vi "Make_Different_Variants_of_Tracks-5.vi"(8 "error IN":errorcluster, 9 "[IN] # of Longest track\nInside the Group of Tracks":i32, 10 "[IN] Index of Earliest \nProblem Point Inside":i32, 11 "[IN] Still connected\ntracks in group":T2) -> (0 "error OUT":errorcluster, 1 "[OUT] Special case!":bool, 3 "[OUT] Subtracks":T1(array[cluster]))   [LabVIEW 2013]
doc: "The subVI formates competing subtracks \nTwo cases are considered: \nSplitting event => only variants after splitting + account the origin of one of subtracks\nMerging event => competition between different variants of elongations"
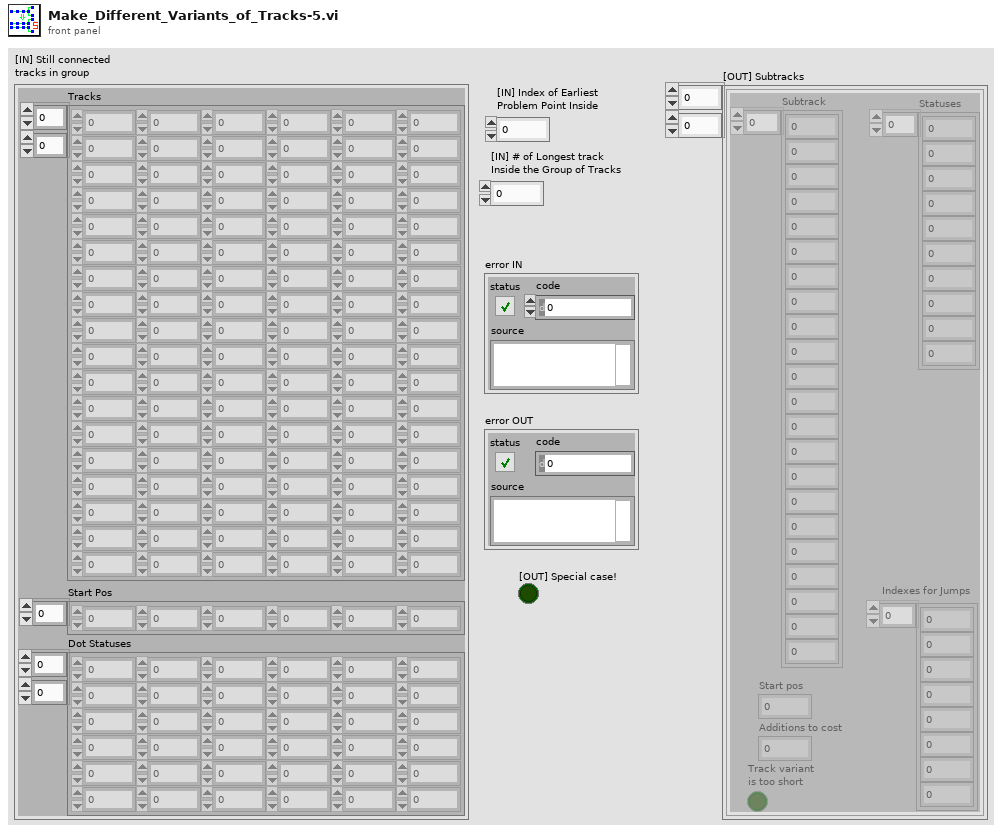
[diagram p1: front panel]
types:
  T1 = cluster{"Subtrack":dbl[], "Statuses":i16[], "Start pos":i32, "Additions to cost":i32, "Track variant \nis too short":bool, "Indexes for Jumps":i32[]}[][]
  T2 = cluster{"Tracks":dbl[][], "Start Pos":i32[], "Dot Statuses":i16[][]}
  T3 = cluster{"Subtrack":dbl[], "Statuses":i16[], "Start pos":i32, "Additions to cost":i32, "Track variant \nis too short":bool, "Indexes for Jumps":i32[]}
  T4 = cluster{"Subtrack":dbl[], "Statuses":i16[], "Start pos":i32, "Additions to cost":i32, "Track variant \nis too short":bool, "Indexes for Jumps":i32[]}[]
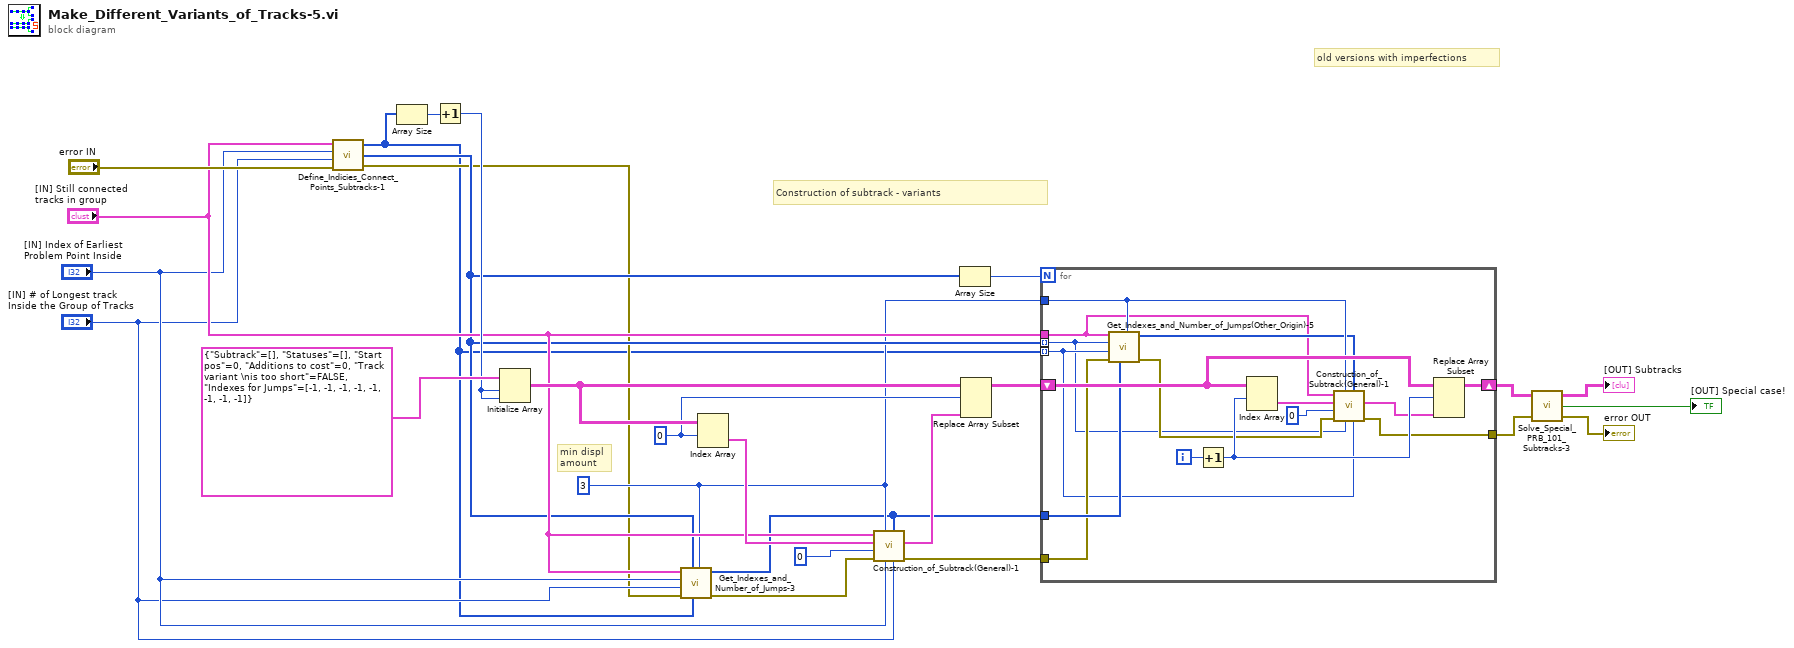
[diagram p0: block diagram]
diagram:
  w20 = 0
  w7 = 3 ("[IN] Minimal Subtrack Length \n(Points without problems) for\nMaking Desicion")
  # "old versions with imperfections"
  # "min displ \namount"
  # "Construction of subtrack - variants"
  n1 = call "Define_Indicies_Connect_Points_Subtracks-1.vi"("error IN"="error IN", "[IN] Index of track with\n(problem displacement)"="[IN] # of Longest track\nInside the Group of Tracks", "[IN] Index of problem\ndisplacement inside track"="[IN] Index of Earliest \nProblem Point Inside", "[IN] Track group"="[IN] Still connected\ntracks in group") -> ("error OUT"=w4:errorcluster, "[OUT] Index of \nconnected dots\ninside the track"=w8:i32[], "[OUT] Index of connected\ntracks with problem dot"=w3:i32[])
  n2 = Array Size(array=w3) -> (size(s)=w25:i32)
  n3 = Increment(x=w25) -> (x+1=w16:i32)
  n4 = Initialize Array(T3 {"Subtrack"=[], "Statuses"=[], "Start pos"=0, "Additions to cost"=0, "Track variant \nis too short"=FALSE, "Indexes for Jumps"=[-1, -1, -1, -1, -1, -1, -1, -1]}, w16, w16) -> (w23:T1)
  n5 = call "Get_Indexes_and_Number_of_Jumps-3.vi"("[IN] Minimal Subtrack\nLength for Making Desicion"=w7, "[IN] Index of connected\ntracks with problem dot"=w3, "[IN] Index of connected \ndots inside the track"=w8, "error IN"=w4, "[IN] # of Track with\nFirst Problem Point"="[IN] # of Longest track\nInside the Group of Tracks", "[IN] Index of First Pro\nblem Point Inside Track"="[IN] Index of Earliest \nProblem Point Inside", "[IN] Still connected\ntracks in group"="[IN] Still connected\ntracks in group") -> ("error OUT"=w2:errorcluster, "[OUT] Indexes for Jumps"=w1:i32[])  [unwired: 1 in, 1 out]
  n6 = Index Array(array=w23, index (row)=w20) -> (element=w22:T4)  [unwired: 1 in]
  n7 = call "Construction_of_Subtrack(General)-1.vi"("[IN] # of Track with\nFirst Problem Point"="[IN] # of Longest track\nInside the Group of Tracks", "[IN] Indexes for Jumps"=w1, "[IN] Index of First Pro\nblem Point Inside Track"="[IN] Index of Earliest \nProblem Point Inside", "[IN] Minimal Subtrack\nLength for Making Desicion"=w7, "error IN"=w2, "[IN] Count of variants"=0, "[IN] Subtracks"=w22, "[IN] Still connected\ntracks in group"="[IN] Still connected\ntracks in group") -> ("error OUT"=w17:errorcluster, "[OUT] Subtracks"=w21:T4)  [unwired: 2 in]
  n8 = Array Size(array=w8) -> (size(s)=w18:i32)
  n9 = Replace Array Subset(array=w23, new element=w21, index (row)=w20) -> (w19:T1)  [unwired: 1 in]
  n10 = for {
    N: w18 -> [_]
    shift-right: [w38] -> w11
    shift-left: w19 -> [w39]
    tunnel: "[IN] Still connected\ntracks in group" -> [w27]
    tunnel: w17 -> [w30]
    tunnel: w8 -> [w28] mode=indexing
    tunnel: w3 -> [w29] mode=indexing
    tunnel: w7 -> [w34]
    tunnel: w1 -> [w33]
    tunnel: [w35] -> w10
    i -> [w42]
    n11 = call "Get_Indexes_and_Number_of_Jumps(Other_Origin)-5.vi"("[IN] Minimal Subtrack\nLength for Making Desicion"=w34, "[IN] Indexes for Jumps\nfrom Previous Origin"=w33, "error IN"=w30, "[IN] # of Track with\nFirst Problem Point"=w29, "[IN] Index of First Pro\nblem Point Inside Track"=w28, "[IN] Still connected\ntracks in group"=w27) -> ("error OUT"=w31:errorcluster, "[OUT] Indexes for Jumps\nFROM new Origin"=w32:i32[])  [unwired: 2 in, 1 out]
    n12 = Increment(x=w42) -> (x+1=w37:i32)
    n13 = Index Array(array=w39, index (row)=w37) -> (element=w41:T4)  [unwired: 1 in]
    n14 = call "Construction_of_Subtrack(General)-1.vi"("[IN] # of Track with\nFirst Problem Point"=w29, "[IN] Indexes for Jumps"=w32, "[IN] Index of First Pro\nblem Point Inside Track"=w28, "[IN] Minimal Subtrack\nLength for Making Desicion"=w34, "error IN"=w31, "[IN] Count of variants"=0, "[IN] Subtracks"=w41, "[IN] Still connected\ntracks in group"=w27) -> ("error OUT"=w35:errorcluster, "[OUT] Subtracks"=w36:T4)  [unwired: 2 in]
    n15 = Replace Array Subset(array=w39, new element=w36, index (row)=w37) -> (w38:T1)  [unwired: 1 in]
  }
  n16 = call "Solve_Special_PRB_101_Subtracks-3.vi"("error IN"=w10, "[IN] Subtracks"=w11) -> ("error OUT"=→"error OUT":errorcluster, "[OUT] Special case!"=→"[OUT] Special case!":bool, "[OUT] Subtracks"=→"[OUT] Subtracks":T1)  [unwired: 1 in]
